vi "Write Atts.vi"(6 "Points":i32, 7 "IF_Band":dbl, 8 "error in (no error)":errorcluster, 9 "Stop":dbl, 10 "Start":dbl, 11 "network in":refnum<class "network.lvclass">) -> (0 "error out":errorcluster, 3 "network out":refnum<class "network.lvclass">)   [LabVIEW 2015, in "network.lvclass"]
uses:
  network.lvclass
  network.lvclass/network.ctl
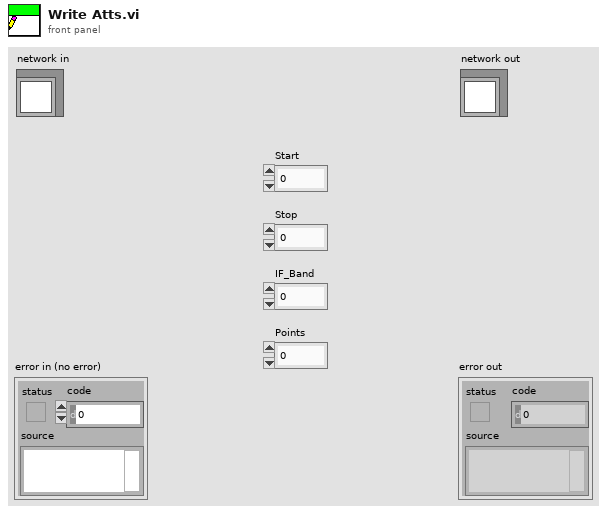
[diagram p1: front panel]
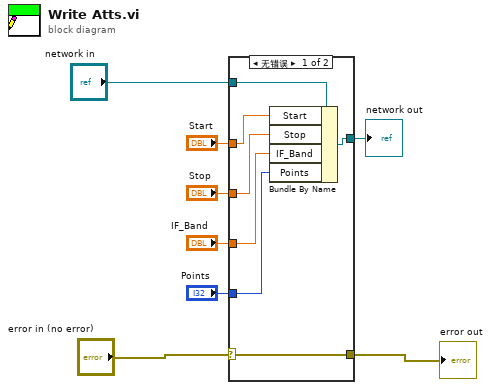
[diagram p0: block diagram]
diagram:
  n1 = case shown="无错误" "error in (no error)" {
    selector: "error in (no error)" -> [w15 w16]
    tunnel: [w15 w16] -> w7
    tunnel: [w13 w17] -> w5
    tunnel: "network in" -> [w14 w17]
    tunnel: "Start" -> [w12 _]
    tunnel: "Points" -> [w11 _]
    tunnel: "IF_Band" -> [w10 _]
    tunnel: "Stop" -> [w9 _]
    frame No Error {
      n2 = Bundle By Name(cluster=w14, "Start"=w12, "Stop"=w9, "IF_Band"=w10, "Points"=w11) -> (w13:refnum<class "network.lvclass">)
    }
    frame Error {
    }
  }
  "error out" <- w7
  "network out" <- w5
